vi "Field Relative Swerve.vi"(8 "Field Relative Active":bool, 11 "Axes Magnitudes":cluster{"X":dbl, "Y":dbl, "Z":dbl}) -> (3 "Axes Mag. Changed":cluster{"X":dbl, "Y":dbl, "Z":dbl})   [LabVIEW 2017, in "Huskie Swerve.lvlib"]
uses:
  Huskie Swerve.lvlib
  Sensors.ctl
  Refname to String (Sensors).vi
  Public/Documents/Cross The Road Electronics/Phoenix-LabVIEW/Pigeon IMU/CTRE_PigeonIMU_GetYPR.vi
  <vilib>/ptbypt/NI_PtbyPt.lvlib
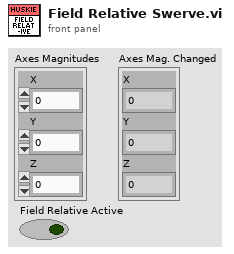
[diagram p1: front panel]
types:
  T1 = typedef "Huskie Swerve.lvlib/Sensors.ctl" = enum16{"Gyro", "Vision USB", "Button Pressed", "Other sensor", "Generic Sensor"}
  T2 = typedef "CTRE_PigeonIMU_DeviceRef.ctl" = cluster{"DeviceStatus":errorcluster, "Device Number":u8, "Type":T3, "Device ID":u32, "Handle":u64, "UsageFrame":u32, "Library Path":path}
  T3 = typedef "CTRE_PigeonIMU_ConnectionType.ctl" = u32
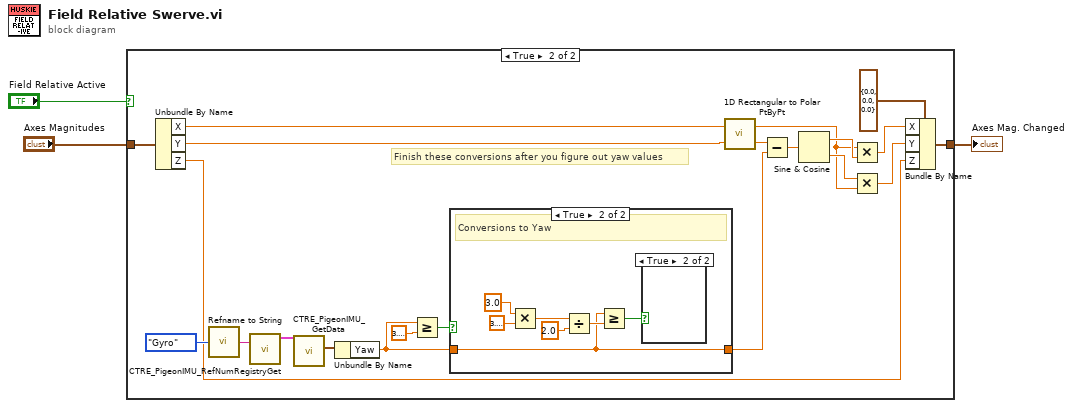
[diagram p0: block diagram]
diagram:
  n1 = case shown="True" "Field Relative Active" {
    tunnel: "Axes Magnitudes" -> [w4 w24]
    tunnel: [w4 w8] -> w2
    frame False {
    }
    frame True {
      # "Finish these conversions after you figure out yaw values"
      n2 = Unbundle By Name(w24) -> ("X"=w23:dbl, "Y"=w22:dbl, "Z"=w9:dbl)
      n3 = call-poly "Refname to String.vi"("Enum"=Sensors."Gyro") -> ("resulting string"=w7:string)
      n4 = call "CTRE_PigeonIMU_RefNumRegistryGet.vi"("refnum name"=w7) -> ("PigeonIMUDevRef"=w6:T2)  [unwired: 9 in, 1 out]
      n5 = call-poly "CTRE_PigeonIMU_GetData.vi"("PigeonIMUDevRef"=w6) -> ("Yaw Pitch Roll"=w5:cluster{"Yaw":dbl, "Pitch":dbl, "Roll":dbl})  [unwired: 8 in, 2 out]
      n6 = Unbundle By Name(w5) -> ("Yaw"=w18:dbl)
      n7 = Greater Or Equal?(x=w18, y=3.141592653589793) -> (x >= y?=w19:bool)
      n8 = case shown="True" w19 {
        tunnel: w18 -> [w26 w28]
        tunnel: [w26 w28] -> w17
        frame False {
        }
        frame True {
          # "Conversions to Yaw"
          n9 = Multiply(x=3.0, y=3.141592653589793) -> (x*y=w31:dbl)
          n10 = Divide(x=w31, y=2.0) -> (x/y=w29:dbl)
          n11 = Greater Or Equal?(x=w28, y=w29) -> (x >= y?=w27:bool)
          n12 = case shown="True" w27 {
            frame False {
            }
            frame True {
            }
          }
        }
      }
      n13 = call <vilib>:"1D Rectangular to Polar PtByPt.vi"("y"=w22, "x"=w23) -> ("phase"=w21:dbl, "magnitude"=w13:dbl)
      n14 = Subtract(x=w21, y=w17) -> (x-y=w16:dbl)
      n15 = Sine & Cosine(0:w16) -> (1:w15:dbl, 2:w14:dbl)
      n16 = Multiply(x=w13, y=w15) -> (x*y=w11:dbl)
      n17 = Multiply(x=w14, y=w13) -> (x*y=w10:dbl)
      n18 = Bundle By Name(cluster=cluster{"X":dbl, "Y":dbl, "Z":dbl} {"X"=0.0, "Y"=0.0, "Z"=0.0} ("Axes Magnitudes 3"), "X"=w11, "Y"=w10, "Z"=w9) -> (w8:cluster{"X":dbl, "Y":dbl, "Z":dbl})
    }
  }
  "Axes Mag. Changed" <- w2
